vi "Disconnect.vi"(8 "error in":errorcluster, 11 "ThorlabsLabJack in":refnum<class "ThorlabsLabJack.lvclass">) -> (0 "error out":errorcluster, 3 "ThorlabsLabJack out":refnum<class "ThorlabsLabJack.lvclass">)   [LabVIEW 2018, in "ThorlabsLabJack.lvlib" / "ThorlabsLabJack.lvclass"]
uses:
  ThorlabsLabJack.lvclass
  ThorlabsLabJack.lvclass/ThorlabsLabJack.ctl
  C:/AME Test Engineering/LabVIEW/PPLs/Axis/Thorlabs/Thorlabs.MotionControl.IntegratedStepperMotorsCLI.dll
  PPLs/Axis/Thorlabs/Thorlabs.MotionControl.IntegratedStepperMotorsCLI.dll
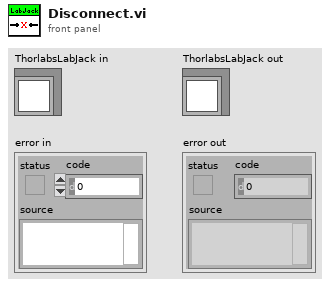
[diagram p1: front panel]
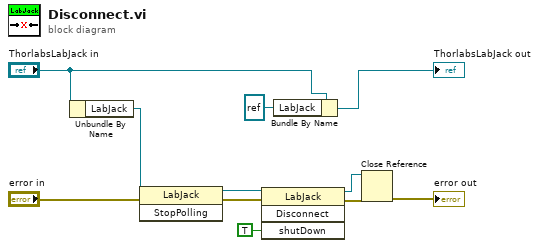
[diagram p0: block diagram]
diagram:
  n1 = Unbundle By Name("ThorlabsLabJack in") -> ("LabJack"=w10:refnum<k24>)
  n2 = invoke class="LabJack" method="StopPolling"(reference=w10, error in="error in") -> (reference out=w9:refnum<k24>, error out=w8:errorcluster)  [unwired: 1 in, 1 out]
  n3 = invoke class="LabJack" method="Disconnect"(reference=w9, error in=w8, "shutDown"=TRUE) -> (reference out=w4:refnum<k24>, error out=w6:errorcluster)  [unwired: 1 in, 2 out]
  n4 = Bundle By Name(cluster="ThorlabsLabJack in", "LabJack"=refnum<k24> refnum) -> (→"ThorlabsLabJack out":refnum<class "ThorlabsLabJack.lvclass">)
  n5 = Close Reference(reference=w4, error in (no error)=w6) -> (error out=→"error out":errorcluster)
